vi "Stage tester - live position.vi"() -> ()   [LabVIEW 2017]
panel:
  in  "stop":bool
  in  "Z":dbl
  in  "Y":dbl
  in  "X":dbl
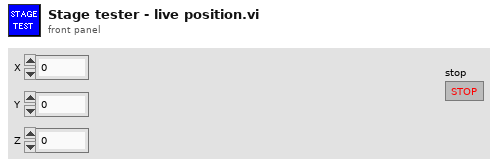
[diagram p1: front panel]
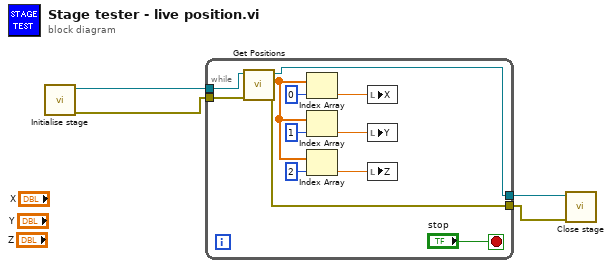
[diagram p0: block diagram]
diagram:
  n1 = call "Initialise stage.vi"() -> ("error out"=w3:errorcluster, "Stage VISA reference"=w2:refnum<visa-resource-name>)  [unwired: 10 in]
  n2 = while {
    tunnel: w3 -> [w15]
    tunnel: [w7] -> w4
    tunnel: w2 -> [w6]
    tunnel: [w5] -> w1
    stop <- "stop" stop-if-true
    n3 = call "Get Positions.vi"("error in"=w15, "Stage VISA in"=w6) -> ("error out"=w7:errorcluster, "Stage current position"=w8:dbl[], "Stage VISA out"=w5:refnum<visa-resource-name>)  [unwired: 7 in]
    n4 = Index Array(array=w8, index=0) -> (element=w13:dbl)
    n5 = Index Array(array=w8, index=1) -> (element=w12:dbl)
    n6 = Index Array(array=w8, index=2) -> (element=w9:dbl)
    n7 = local write "X"(w13) -> ()
    n8 = local write "Y"(w12) -> ()
    n9 = local write "Z"(w9) -> ()
  }
  n10 = call "Close stage.vi"("error in"=w4, "VISA resource name"=w1) -> ()  [unwired: 9 in, 1 out]
